vi "DSF.Engine.BuilderManager.Get Builders.vi"(11 "Builder Manager in":refnum<class "DSF.Engine.BuilderManager.lvclass">) -> (2 "Builders":refnum<class "DSF.Engine.Builder.lvclass">[](array[class]), 3 "Builder Manager out":refnum<class "DSF.Engine.BuilderManager.lvclass">)   [LabVIEW 2017, in "DSF.Engine.lvlib" / "DSF.Engine.BuilderManager.lvclass"]
uses:
  DSF.Engine.BuilderManager.lvclass
  Builder/DSF.Engine.Builder.lvclass
  DSF.Engine.BuilderManager.lvclass/DSF.Engine.BuilderManager.ctl
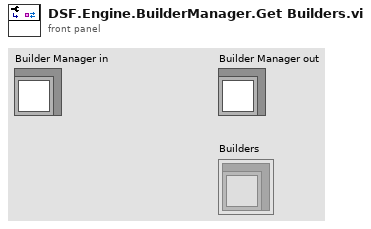
[diagram p1: front panel]
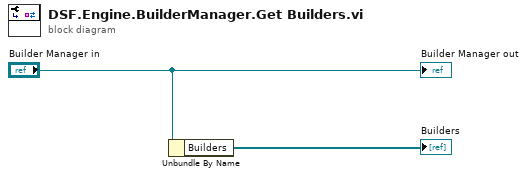
[diagram p0: block diagram]
diagram:
  n1 = Unbundle By Name("Builder Manager in") -> ("Builders"=→"Builders":refnum<class "DSF.Engine.Builder.lvclass">[])
  "Builder Manager out" <- "Builder Manager in"
